vi "Create Temporary File Path.vi"(4 "error in":errorcluster, 6 "filename":string="temp.tmp") -> (0 "error out":errorcluster, 3 "filepath":path)   [LabVIEW 2010]
doc: "Returns a unique file path to the temporary directory. This VI only returns a path. It does not create the temporary file."
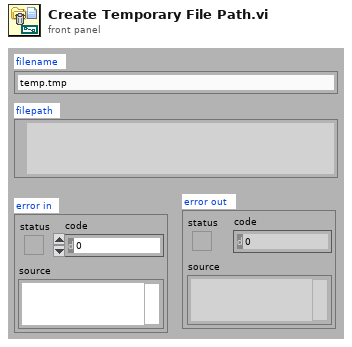
[diagram p1: front panel]
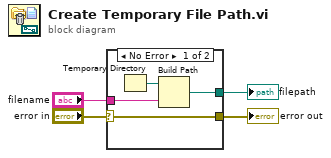
[diagram p0: block diagram]
diagram:
  n1 = case shown="No Error" "error in" {
    selector: "error in" -> [w6 w9]
    tunnel: "filename" -> [w7 _]
    tunnel: [w5 _] -> w2
    tunnel: [w6 w9] -> w1
    frame No Error {
      n2 = Temporary Directory() -> (w8:path)
      n3 = Build Path(base path=w8, name or relative path=w7) -> (appended path=w5:path)
    }
    frame Error {
    }
  }
  "error out" <- w1
  "filepath" <- w2
